vi "check if brackets Matched 2.vi"(11 "regular expression":string="[{String:abc;BoolArray:[TRUE,FALSE,TRUE,FALSE]},{String:def;BoolArray:[FALSE,TRUE,FALSE,TRUE]},{String:xyz;BoolArray:[TRUE,TRUE,FALSE,FALSE]}]") -> (0 "Matched?":bool=TRUE, 3 "regular expression (dup)":string="[{String:abc;BoolArray:[TRUE,FALSE,TRUE,FALSE]},{String:def;BoolArray:[FALSE,TRUE,FALSE,TRUE]},{String:xyz;BoolArray:[TRUE,TRUE,FALSE,FALSE]}]")   [LabVIEW 2017, in "API String Arguments Support.lvlib"]
uses:
  API String Arguments Support.lvlib
  <userlib>/_NEVSTOP/Communicable State Machine(CSM)/Communicable State Machine.lvlib
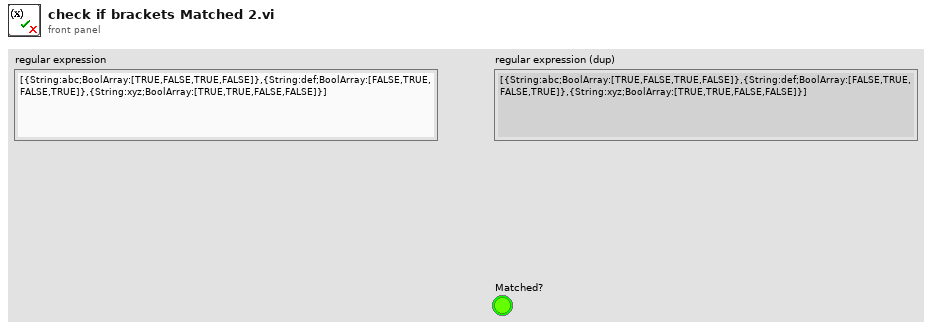
[diagram p1: front panel]
types:
  T1 = enum16{"0x2829 - ()", "0x5B5D - []", "0x7B7D - {}"}
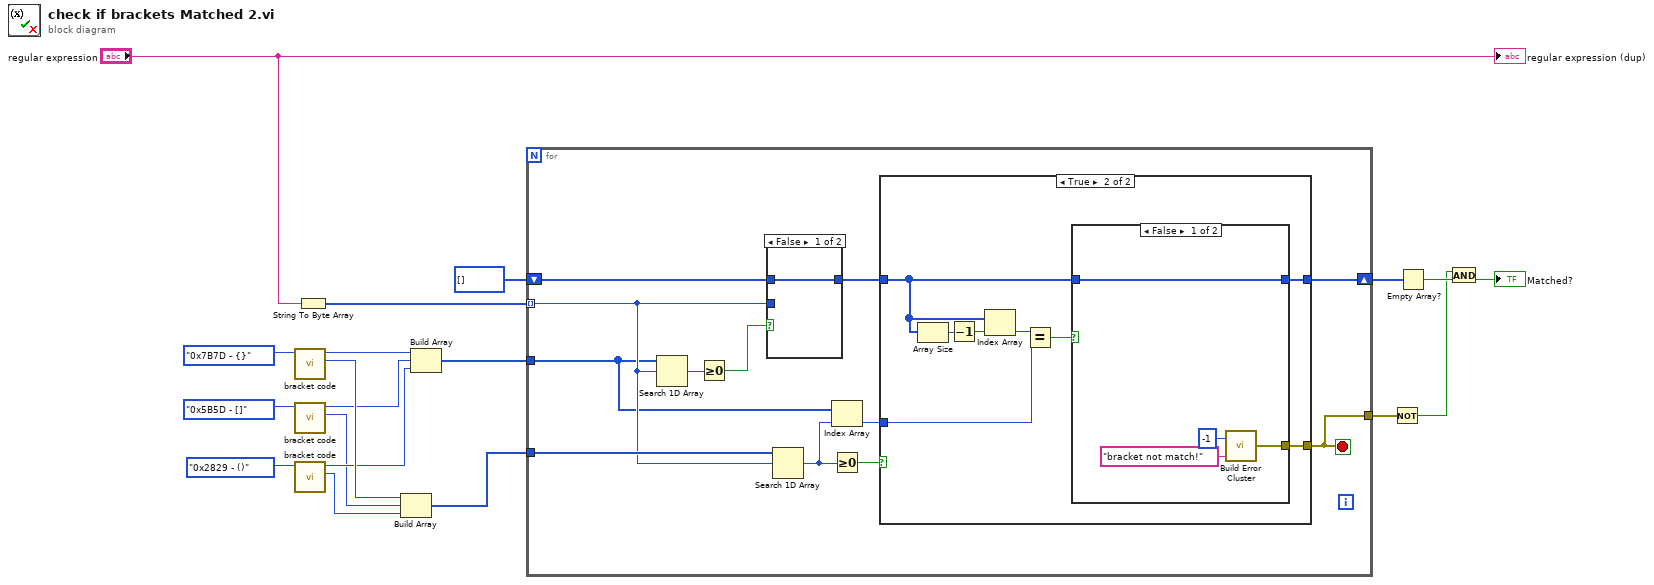
[diagram p0: block diagram]
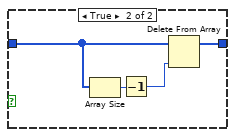
[diagram p3: hidden frame]
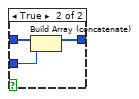
[diagram p4: hidden frame]
diagram:
  n1 = call "bracket code.vi"("Enum"=T1."0x7B7D - {}" ("TYPE")) -> ("Numeric"=w11:u8, "Numeric 2"=w15:u8)  [unwired: 9 in]
  n2 = call "bracket code.vi"("Enum"=T1."0x5B5D - []" ("TYPE")) -> ("Numeric"=w8:u8, "Numeric 2"=w10:u8)  [unwired: 9 in]
  n3 = call "bracket code.vi"("Enum"=T1."0x2829 - ()" ("TYPE")) -> ("Numeric"=w7:u8, "Numeric 2"=w9:u8)  [unwired: 9 in]
  n4 = String To Byte Array(string="regular expression") -> (unsigned byte array=w17:u8[])
  n5 = Build Array(w11, w8, w7) -> (w6:u8[])
  n6 = Build Array(w15, w10, w9) -> (w12:u8[])
  n7 = for {
    tunnel: w17 -> [w24] mode=indexing
    shift-right: [w29] -> w4
    shift-left: u8[] [] -> [w30]
    tunnel: w12 -> [w22]
    tunnel: w6 -> [w26]
    tunnel: [w20] -> w2
    stop <- w20 stop-if-true
    n8 = Search 1D Array(1D array=w22, element=w24) -> (index of element=w28:i32)  [unwired: 1 in]
    n9 = Greater Or Equal To 0?(x=w28) -> (x >= 0?=w27:bool)
    n10 = case shown="False" w27 {
      tunnel: w30 -> [w49 w52]
      tunnel: w24 -> [_ w51]
      tunnel: [w49 w50] -> w31
      frame False {
      }
      frame True {
        n11 = Build Array (concatenate)(w52, w51) -> (w50:u8[])
      }
    }
    n12 = Search 1D Array(1D array=w26, element=w24) -> (index of element=w21:i32)  [unwired: 1 in]
    n13 = Index Array(array=w22, index=w21) -> (element=w23:u8)
    n14 = Greater Or Equal To 0?(x=w21) -> (x >= 0?=w25:bool)
    n15 = case shown="True" w25 {
      tunnel: w31 -> [w32 w37]
      tunnel: [w32 w40] -> w29
      tunnel: w23 -> [_ w35]
      tunnel: [_ w33] -> w20
      frame False {
      }
      frame True {
        n16 = Array Size(array=w37) -> (size(s)=w39:i32)
        n17 = Decrement(x=w39) -> (x-1=w38:i32)
        n18 = Index Array(array=w37, index=w38) -> (element=w36:u8)
        n19 = Equal?(x=w36, y=w35) -> (x = y?=w34:bool)
        n20 = case shown="False" w34 {
          tunnel: w37 -> [w44 w47]
          tunnel: [w44 w45] -> w40
          tunnel: [w41 _] -> w33
          frame False {
            n21 = call <userlib>:"Build Error Cluster.vi"("String to Prepend to source (\"\")"="bracket not match!" ("String to Prepend to source (\"\")"), "code"=-1) -> ("error out"=w41:errorcluster)
          }
          frame True {
            n22 = Array Size(array=w47) -> (size(s)=w48:i32)
            n23 = Decrement(x=w48) -> (x-1=w46:i32)
            n24 = Delete From Array(array=w47, index=w46) -> (array with subset deleted=w45:u8[])  [unwired: 1 in, 1 out]
          }
        }
      }
    }
  }
  n25 = Not(x=w2) -> (.not. x?=w1:bool)
  n26 = Empty Array?(array=w4) -> (empty?=w19:bool)
  n27 = And(x=w1, y=w19) -> (x .and. y?=→"Matched?":bool)
  "regular expression (dup)" <- "regular expression"
